vi "Migrate Global Config.vi"(8 "error in (no error)":errorcluster, 10 "Old Global Config":path, 11 "App Data Directory":path) -> (0 "error out":errorcluster)   [LabVIEW 2020, in "MacroAssert.lvlib"]
doc: "Migrates any old global configuration data from the old location to the new location."
uses:
  MacroAssert.lvlib
  CTLs/Hotkey Type.ctl
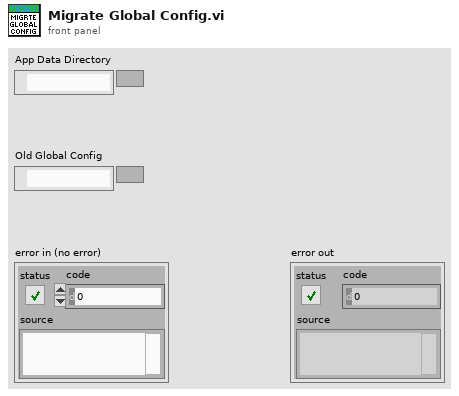
[diagram p1: front panel]
types:
  T1 = typedef "MacroAssert.lvlib/Hotkey Type.ctl" = enum16{"Macro Hotkey", "Abort Hotkey"}
  T2 = typedef "MacroAssert.lvlib/Hotkey Values.ctl" = cluster{"Macro Hotkey":enum16{"0", "1", "2", "3", "4", "5", "6", "7", "8", "9", "A", "B", "C", "D", "E", "F", "G", "H", "I", "J", "K", "L", "M", "N", "O", "P", "Q", "R", "S", "T", "U", "V", "W", "X", "Y", "Z", "F1", "F2", "F3", "F4", "F5", "F6", "F7", "F8", "F9", "F10", "F11", "F12", "F13", "F14", "F15", "ADD", "BACK", "BACKSLASH", "CAPITAL", "COMMA", "DECIMAL", "DELETE", "DIVIDE", "DOWN", "END", "EQUALS", "ESCAPE", "GRAVE (`)", "HOME", "INSERT", "LBRACKET", "LCONTROL", "LEFT", "L ALT", "LSHIFT", "LWIN", "MINUS", "MULTIPLY", "NEXT", "NUMLOCK", "NUMPAD_0", "NUMPAD_1", "NUMPAD_2", "NUMPAD_3", "NUMPAD_4", "NUMPAD_5", "NUMPAD_6", "NUMPAD_7", "NUMPAD_8", "NUMPAD_9", "PAUSE", "PERIOD", "PRIOR (PG UP)", "RBRACKET", "RCONTROL", "RETURN", "RIGHT", "R ALT", "RSHIFT", "RWIN", "SCROLL", "SEMICOLON", "SLASH", "SPACE", "SUBTRACT", "TAB", "UP", "ENTER (num pad)", "' (quote)"}[], "Abort Hotkey":enum16{"0", "1", "2", "3", "4", "5", "6", "7", "8", "9", "A", "B", "C", "D", "E", "F", "G", "H", "I", "J", "K", "L", "M", "N", "O", "P", "Q", "R", "S", "T", "U", "V", "W", "X", "Y", "Z", "F1", "F2", "F3", "F4", "F5", "F6", "F7", "F8", "F9", "F10", "F11", "F12", "F13", "F14", "F15", "ADD", "BACK", "BACKSLASH", "CAPITAL", "COMMA", "DECIMAL", "DELETE", "DIVIDE", "DOWN", "END", "EQUALS", "ESCAPE", "GRAVE (`)", "HOME", "INSERT", "LBRACKET", "LCONTROL", "LEFT", "L ALT", "LSHIFT", "LWIN", "MINUS", "MULTIPLY", "NEXT", "NUMLOCK", "NUMPAD_0", "NUMPAD_1", "NUMPAD_2", "NUMPAD_3", "NUMPAD_4", "NUMPAD_5", "NUMPAD_6", "NUMPAD_7", "NUMPAD_8", "NUMPAD_9", "PAUSE", "PERIOD", "PRIOR (PG UP)", "RBRACKET", "RCONTROL", "RETURN", "RIGHT", "R ALT", "RSHIFT", "RWIN", "SCROLL", "SEMICOLON", "SLASH", "SPACE", "SUBTRACT", "TAB", "UP", "ENTER (num pad)", "' (quote)"}[]}
  T3 = enum16{"0", "1", "2", "3", "4", "5", "6", "7", "8", "9", "A", "B", "C", "D", "E", "F", "G", "H", "I", "J", "K", "L", "M", "N", "O", "P", "Q", "R", "S", "T", "U", "V", "W", "X", "Y", "Z", "F1", "F2", "F3", "F4", "F5", "F6", "F7", "F8", "F9", "F10", "F11", "F12", "F13", "F14", "F15", "ADD", "BACK", "BACKSLASH", "CAPITAL", "COMMA", "DECIMAL", "DELETE", "DIVIDE", "DOWN", "END", "EQUALS", "ESCAPE", "GRAVE (`)", "HOME", "INSERT", "LBRACKET", "LCONTROL", "LEFT", "L ALT", "LSHIFT", "LWIN", "MINUS", "MULTIPLY", "NEXT", "NUMLOCK", "NUMPAD_0", "NUMPAD_1", "NUMPAD_2", "NUMPAD_3", "NUMPAD_4", "NUMPAD_5", "NUMPAD_6", "NUMPAD_7", "NUMPAD_8", "NUMPAD_9", "PAUSE", "PERIOD", "PRIOR (PG UP)", "RBRACKET", "RCONTROL", "RETURN", "RIGHT", "R ALT", "RSHIFT", "RWIN", "SCROLL", "SEMICOLON", "SLASH", "SPACE", "SUBTRACT", "TAB", "UP", "ENTER (num pad)", "' (quote)"}[]
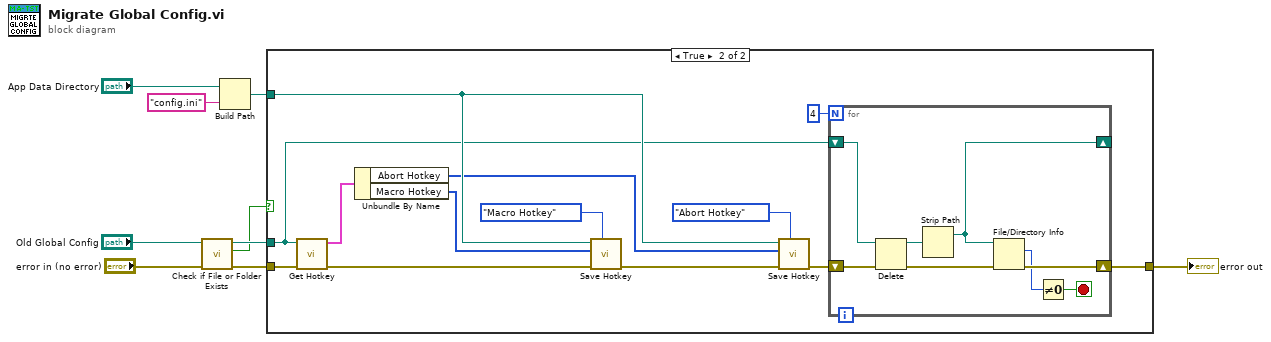
[diagram p0: block diagram]
diagram:
  n1 = call <vilib>:"Check if File or Folder Exists.vi"("error in (no error)"="error in (no error)", "path"="Old Global Config") -> ("error out"=w7:errorcluster, "file or folder exists?"=w4:bool, "dup path"=w8:path)  [unwired: 7 in]
  n2 = Build Path(base path="App Data Directory", name or relative path="config.ini") -> (appended path=w2:path)
  n3 = case shown="True" w4 {
    tunnel: w8 -> [_ w11]
    tunnel: w7 -> [w10 w23]
    tunnel: w2 -> [_ w19]
    tunnel: [w10 w13] -> w5
    frame False {
    }
    frame True {
      n4 = call "Get Hotkey.vi"("error in (no error)"=w23, "File Path"=w11) -> ("error out"=w22:errorcluster, "Hotkey Values"=w21:T2)  [unwired: 8 in]
      n5 = Unbundle By Name(w21) -> ("Abort Hotkey"=w15:T3, "Macro Hotkey"=w16:T3)
      n6 = call "Save Hotkey.vi"("Hotkey Type"=Hotkey_Type."Macro Hotkey", "error in (no error)"=w22, "Hotkey"=w16, "File Path"=w19) -> ("error out"=w20:errorcluster)  [unwired: 7 in]
      n7 = call "Save Hotkey.vi"("Hotkey Type"=Hotkey_Type."Abort Hotkey", "error in (no error)"=w20, "Hotkey"=w15, "File Path"=w19) -> ("error out"=w14:errorcluster)  [unwired: 7 in]
      n8 = for {
        N: 4 -> [_]
        shift-right: [w24] -> _
        shift-left: w11 -> [w30]
        shift-right: [w27] -> w13
        shift-left: w14 -> [w31]
        stop <- w25 stop-if-true
        n9 = Delete(path (use dialog)=w30, error in=w31) -> (deleted path=w29:path, error out=w28:errorcluster)  [unwired: 3 in, 1 out]
        n10 = Strip Path(path=w29) -> (stripped path=w24:path)  [unwired: 1 out]
        n11 = File/Directory Info(path=w24, error in=w28) -> (size=w26:i64, error out=w27:errorcluster)  [unwired: 5 out]
        n12 = Not Equal To 0?(x=w26) -> (x != 0?=w25:bool)
      }
    }
  }
  "error out" <- w5
